vi "Build the ppl.vi"(11 "Command line args":string[](array[string])) -> (2 "Output/Error messages":string, 3 "CLI Process Return Code":i32)   [LabVIEW 2021]
uses:
  <vilib>/AppBuilder/AB_API_Simple/Build (path).vi
  <vilib>/AppBuilder/AB_API_Simple/NI_App_Builder_API.lvlib
panel:
  out "Generated files":path[](array[path])
  out "error out":errorcluster
  in  "error in (no error)":errorcluster
  in  "Name of target (My Computer)":string="My Computer"
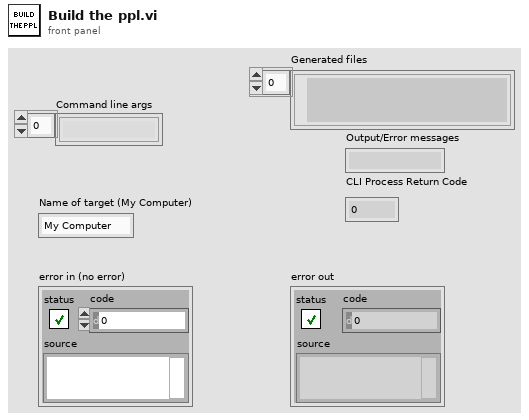
[diagram p1: front panel]
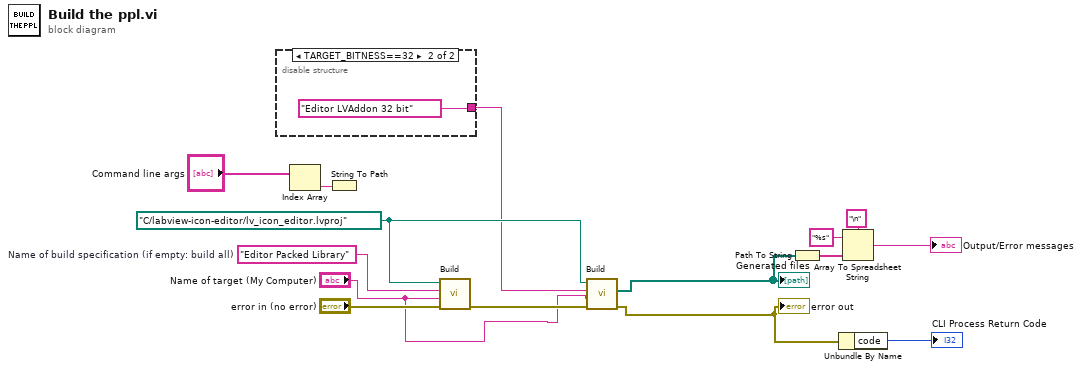
[diagram p0: block diagram]
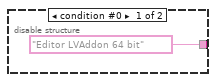
[diagram p2: hidden frame]
diagram:
  w5 = path "C:/labview-icon-editor/lv_icon_editor.lvproj" ("Path override")
  w15 = "Editor Packed Library"  # Name of build specification (if empty: build all)
  n1 = disable-structure shown="TARGET_BITNESS==32" {
    disable-tunnel: ["Editor LVAddon 64 bit" ("Name of build specification (if empty: build all)") "Editor LVAddon 32 bit" ("Name of build specification (if empty: build all)")] -> w1
    frame condition #0 {
    }
    frame condition #1 (active) {
    }
  }
  n2 = Index Array(array="Command line args") -> (element=w12:string)  [unwired: 1 in]
  n3 = String To Path(string=w12) -> ()  [unwired: 1 out]
  n4 = call-poly <vilib>:"Build.vi"("error in (no error)"="error in (no error)", "Name of target (My Computer)"="Name of target (My Computer)", "Name of build specification (if empty: build all)"=w15, "Path to project"=w5) -> ("error out"=w6:errorcluster)  [unwired: 6 in, 1 out]
  n5 = call-poly <vilib>:"Build.vi"("error in (no error)"=w6, "Name of target (My Computer)"="Name of target (My Computer)", "Name of build specification (if empty: build all)"=w1, "Path to project"=w5) -> ("error out"=w3:errorcluster, "Generated files"=w4:path[])  [unwired: 6 in]
  "error out" <- w3
  "Generated files" <- w4
  n6 = Path To String(path=w4) -> (string=w11:string[])
  n7 = Unbundle By Name(w3) -> ("code"=→"CLI Process Return Code":i32)
  n8 = Array To Spreadsheet String(delimiter (Tab)="\n", array=w11, 3:"%s" ("format string")) -> (spreadsheet string=→"Output/Error messages":string)
